vi "Multiple Chassis Synchronization - Scopes Synchronized with TCLK.vi"() -> ()   [LabVIEW 2026]
uses:
  SubVIs/NI SYNC Abstraction/Lib/Trigger Routing.ctl
  SubVIs/NI SYNC Abstraction/Lib/Clock Routing.ctl
  <instrlib>/niScope/Controls/niScope export destinations.ctl
  Types/MyState.ctl
  <instrlib>/niScope/Controls/niScope input clock source.ctl
  Types/MyVariables.ctl
  <instrlib>/niScope/Controls/niScope exportable signals.ctl
  <instrlib>/niFgen/niFgen.llb/niFgen Output Mode.ctl
  <instrlib>/niScope/Configure/Trigger/niScope Configure Trigger Edge.vi
  <instrlib>/niScope/Configure/Trigger/niScope Configure Trigger Digital.vi
  <instrlib>/niSync/niSync.llb/niSync Initialize (IVI).vi
  SubVIs/NI SYNC Abstraction/Lib/Connect Clock Terminals-Array.vi
  SubVIs/NI SYNC Abstraction/Lib/Connect Clock Terminals.vi
  SubVIs/NI SYNC Abstraction/Lib/Connect Trigger Terminals-Array.vi
  SubVIs/NI SYNC Abstraction/Lib/Connect Trigger Terminals.vi
  SubVIs/NI SYNC Abstraction/Lib/Disonnect Trigger Terminals-Array.vi
  SubVIs/NI SYNC Abstraction/Lib/Disonnect Trigger Terminals.vi
  <instrlib>/niScope/Acquire/Fetch/niScope Fetch Cluster.vi
  SubVIs/NI SYNC Abstraction/Lib/Disconnect Clock Terminals-Array.vi
  SubVIs/NI SYNC Abstraction/Lib/Disconnect Clock Terminals.vi
  <resource>/objmgr/sessionReference.rc
  <vilib>/ptbypt/NI_PtbyPt.lvlib
panel:
  in  "Tab Control":T1(tab)
  in  "Master.Scope":refnum<k15>="PXI1_SCOPE1"
  in  "Rest.Scopes":refnum<k15>[](array[refnum])=["PXI2_SCOPE2"]
  in  "Master.6674T_1":refnum<k15>="PXI1_MasterSync"
  in  "Rest.6674T_1":refnum<k15>="PXI2_SlaveSync"
  in  "FGEN.Ref":refnum<k15>="PXI1_FGEN1"
  in  "Routing":T2(tab)
  in  "Rest.In --> Clk10":T3={"Source Terminal"="ClkIn", "Destination Terminal"="PXI_Clk10_In"}
  in  "Master.In --> Clk10":T3={"Source Terminal"="ClkIn", "Destination Terminal"="PXI_Clk10_In"}
  in  "Master.Clock --> Out":T3={"Source Terminal"="Oscillator", "Destination Terminal"="ClkOut"}
  in  "Rest.PFI --> Ref Trigger":T4={"Source"="PFI0", "Destination"="PXI_Trig0", "Synchronization Clock"="SyncClkAsync"}
  in  "Master.Ref Trigger --> PFI":T4={"Source"="PXI_Trig0", "Destination"="PFI0", "Synchronization Clock"="SyncClkAsync"}
  in  "Master.Ref Trigger Export":T5="VAL_RTSI_0"
  in  "Rest.Ref Trigger Source":T5="VAL_RTSI_0"
  in  "Rest.Start Trigger Source":T5="VAL_RTSI_1"
  in  "Rest.PFI --> Start Trigger":T4={"Source"="PFI1", "Destination"="PXI_Trig1", "Synchronization Clock"="SyncClkAsync"}
  in  "Master.Start Trigger --> PFI":T4={"Source"="PXI_Trig1", "Destination"="PFI2", "Synchronization Clock"="SyncClkAsync"}
  in  "Master.Start Trigger Export":T5="VAL_RTSI_1"
  in  "Rest.Sync Pulse Source":string(combo)="PXI_Trig2"
  in  "Rest.PFI --> Sync Pulse Source":T4={"Source"="PFI1", "Destination"="PXI_Trig2", "Synchronization Clock"="SyncClkAsync"}
  in  "Master.PFI --> Sync Pulse Source":T4={"Source"="PFI1", "Destination"="PXI_Trig2", "Synchronization Clock"="SyncClkAsync"}
  in  "Master.Sync Pulse Export --> PFI":T4={"Source"="PXI_Trig3", "Destination"="PFI2", "Synchronization Clock"="SyncClkFullSpeed"}
  in  "Master.Sync Pulse Export":string(combo)="PXI_Trig3"
  in  "Master.Sync Pulse Source":string(combo)="PXI_Trig2"
  in  "Enable Cal?":bool
  in  "Calibration Iterations":i32=10
  in  "Scope 2 tCLK Delay":dbl format="%#_13p"
  in  "Scope 1 tCLK Delay":dbl format="%#_13p"
  out "Cal Iteration Delays":dbl[](array[numeric]) format="%#_p"
  out "Average Delay":dbl format="%.5p"
  out "Standard Deviation":dbl format="%0.2p"
  out "Waveform Graph":T6(graph)
  out "Sample Offset":dbl
  out "error out":errorcluster
  out "Offset Time (s)":dbl format="%#_p"
  # "Scope"
  # "Sync"
  # "Master"
  # "Ref Trigger Export"
  # "Start Trigger Export"
  # "Sync Pulse Source"
  # "Sync Pulse Export"
  # "Sync"
  # "Scope"
  # "Rest"
  # "Ref Trigger Source"
  # "Start Trigger Source"
  # "Sync Pulse Source"
  # "None"
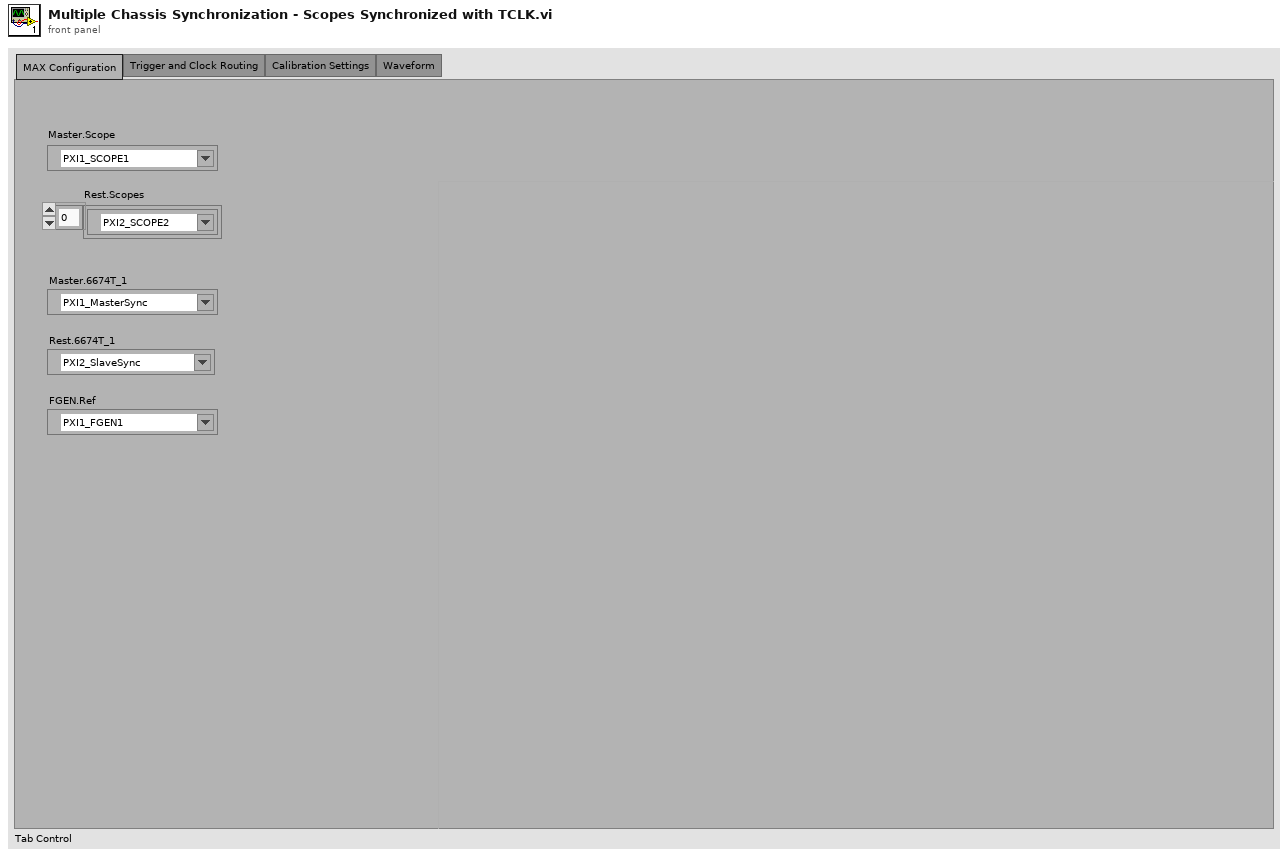
[diagram p1: front panel]
types:
  T1 = enum32{"MAX Configuration", "Trigger and Clock Routing", "Calibration Settings", "Waveform"}
  T2 = enum32{"Clock Routing", "Reference Trigger", "Start Trigger", "Sync Pulse"}
  T3 = typedef "Clock Routing.ctl" = cluster{"Source Terminal":string, "Destination Terminal":string}
  T4 = typedef "Trigger Routing.ctl" = cluster{"Source":string, "Destination":string, "Synchronization Clock":string}
  T5 = typedef "niScope export destinations.ctl" = string
  T6 = cluster{"relativeInitialX":dbl, "xIncrement":dbl, "wfm":dbl[]}[]
  T7 = typedef "MyState.ctl" = enum16{"Initialize", "SCOPE: Config.Master", "SCOPE: Config.Rest", "SYNC: Device.Init", "SYNC: ConnectClock.Master", "SYNC: ConnectClock.Rest", "SYNC: ConnectSyncPulse.Master", "SYNC: ConnectSyncPulse.Rest", "SYNC: ConnectRefTrigger.Master", "SYNC: ConnectRefTrigger.Rest", "TCLK: Config.Master", "TCLK: Config.Rest", "TCLK: ApplyManualCalibration", "TCLK: SendSyncPulse", "SYNC: DisconnectSyncPulse.Master", "SYNC: DisconnectSyncPulse.Rest", "SYNC: ConnectStartTrigger.Master", "SYNC: ConnectStartTrigger.Rest", "TCLK: Commit", "FGEN: StartSquareWave", "SCOPE: Acquire", "FGEN: StopSquareWave", "SYNC: DisconnectStartTrigger.Master", "SYNC: DisconnectStartTrigger.Rest", "SYNC: DisconnectRefTrigger.Master", "SYNC: DisconnectRefTrigger.Rest", "SYNC: DisconnectClock.Master", "SYNC: DisconnectClock.Rest", "Shutdown"}
  T8 = typedef "MyVariables.ctl" = cluster{"Master":cluster{"TimeSync.Ref":refnum<k15>, "TCLK.Ref":refnum<k20>, "Clock":cluster{"Clock --> Out":T3, "In --> Clk10":T3}, "Sync Pulse":cluster{"Sync Pulse Export":string, "Sync Pulse Export --> PFI":T4, "PFI --> Sync Pulse Source":T4, "Sync Pulse Source":string}, "Start Trigger":cluster{"Start Trigger Export":T5, "Start Trigger --> PFI":T4}, "Scope.Ref":refnum<k15>, "Ref Trigger":cluster{"Ref Trigger Export":T5, "Ref Trigger --> PFI":T4}}, "Rest":cluster{"TimeSync.Ref":refnum<k15>, "TCLK.Refs":refnum<k20>[], "Clock":cluster{"In --> Clk10":T3}, "Sync Pulse":cluster{"PFI --> Sync Pulse Source":T4, "Sync Pulse Source":string}, "Start Trigger":cluster{"PFI --> Start Trigger":T4, "Start Trigger Source":T5}, "Scope.Refs":refnum<k15>[], "Ref Trigger":cluster{"PFI --> Ref Trigger":T4, "Ref Trigger Source":T5}}, "FGEN.Ref":refnum<k15>}
  T9 = typedef "niScope input clock source.ctl" = u16
  T10 = typedef "niScope exportable signals.ctl" = u16
  T11 = typedef "niFgen Output Mode.ctl" = u32
  T12 = cluster{"relativeInitialX":dbl, "xIncrement":dbl, "wfm":dbl[]}
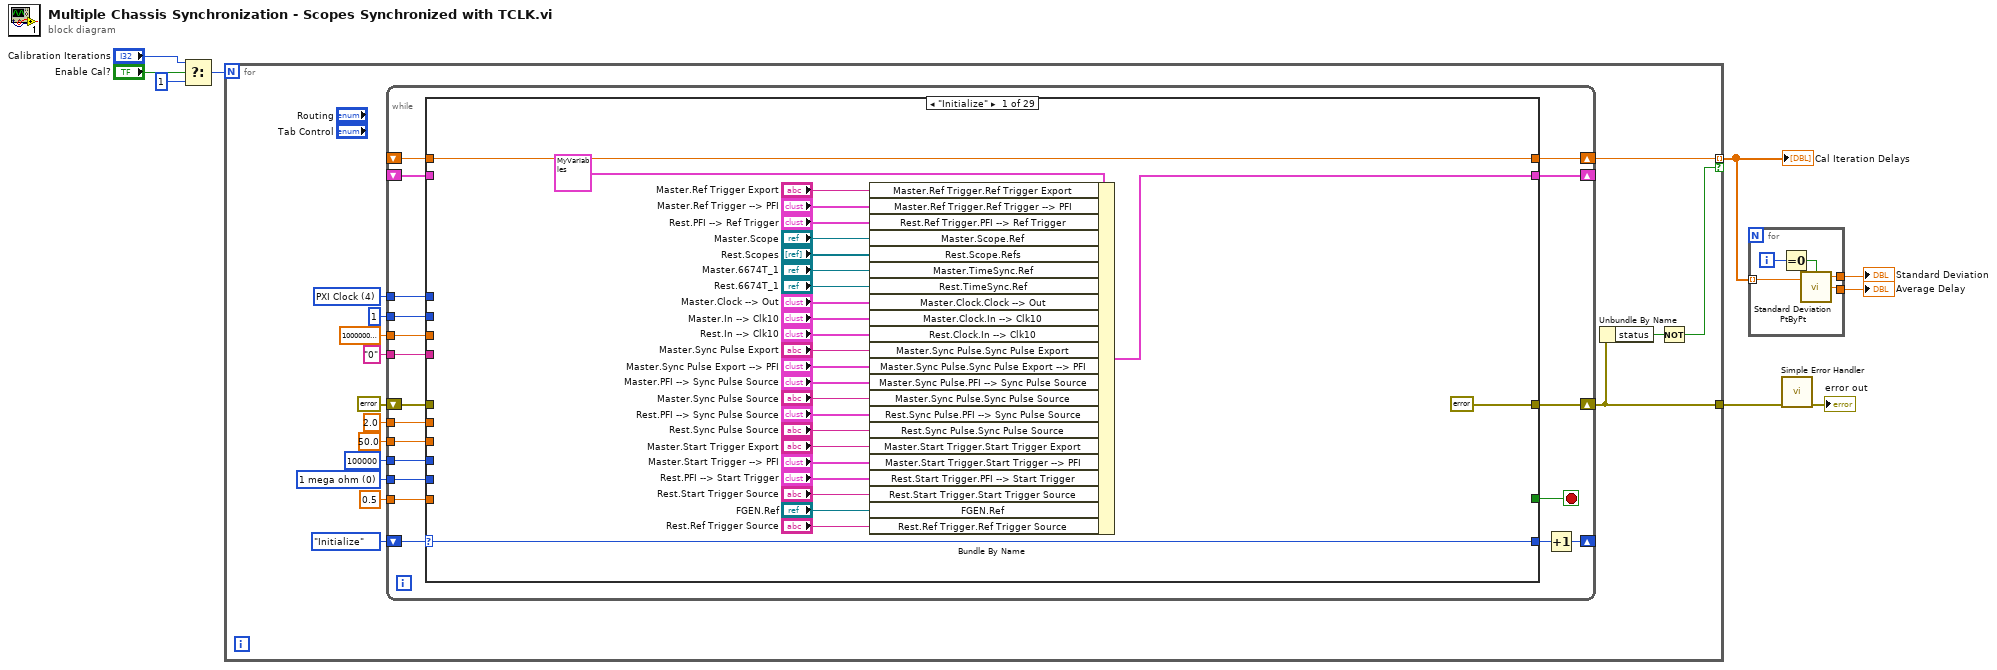
[diagram p0: block diagram]
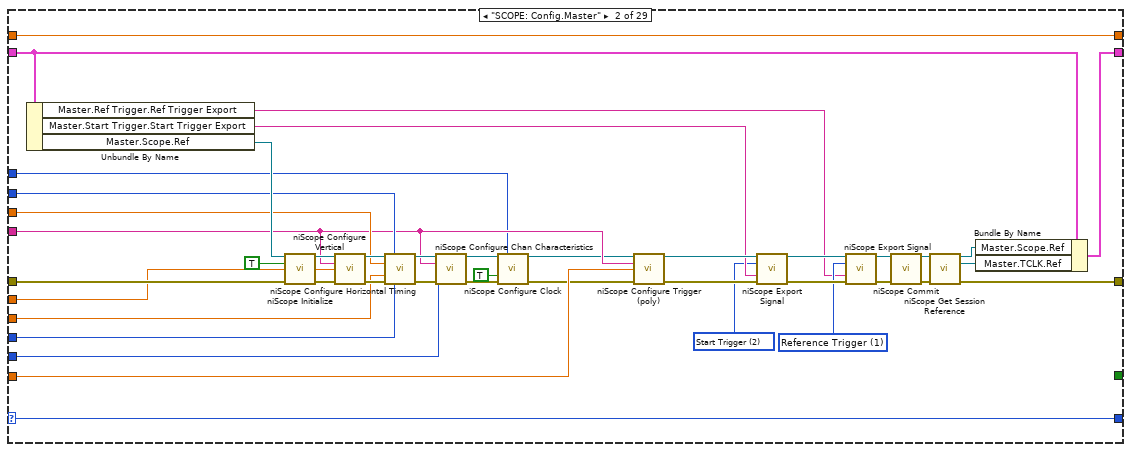
[diagram p2: hidden frame]
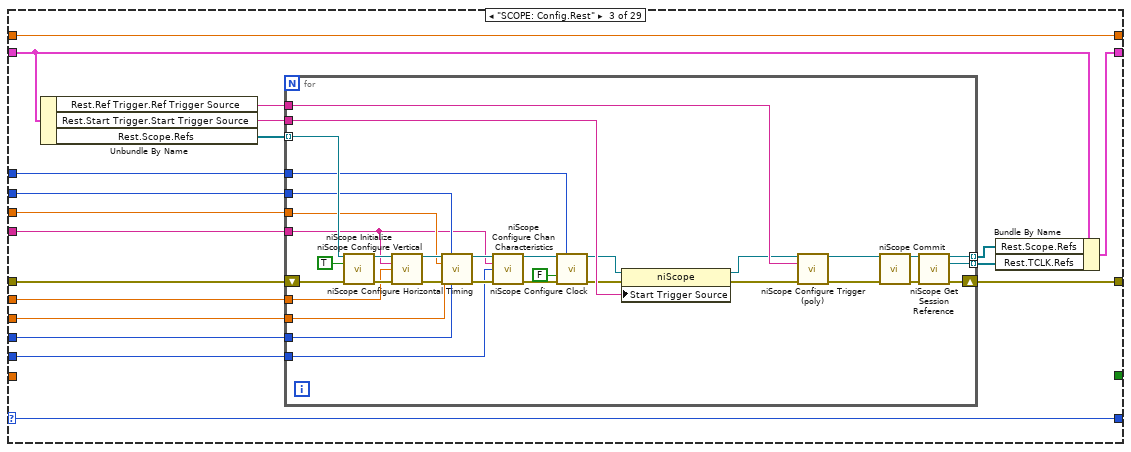
[diagram p3: hidden frame]
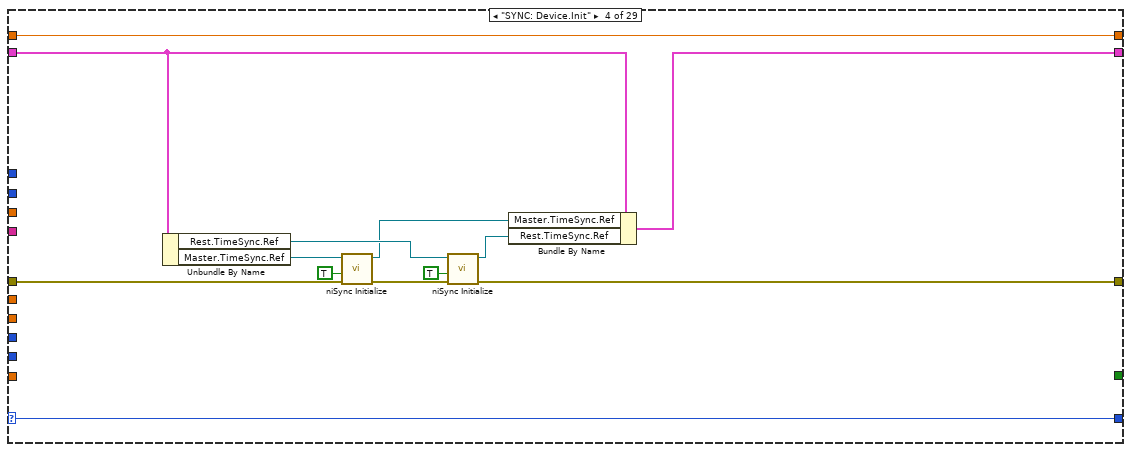
[diagram p4: hidden frame]
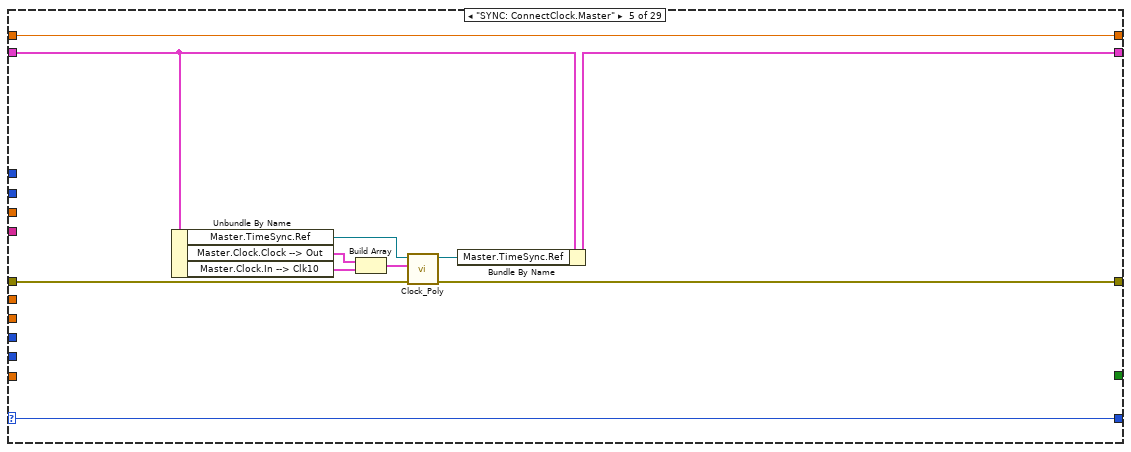
[diagram p5: hidden frame]
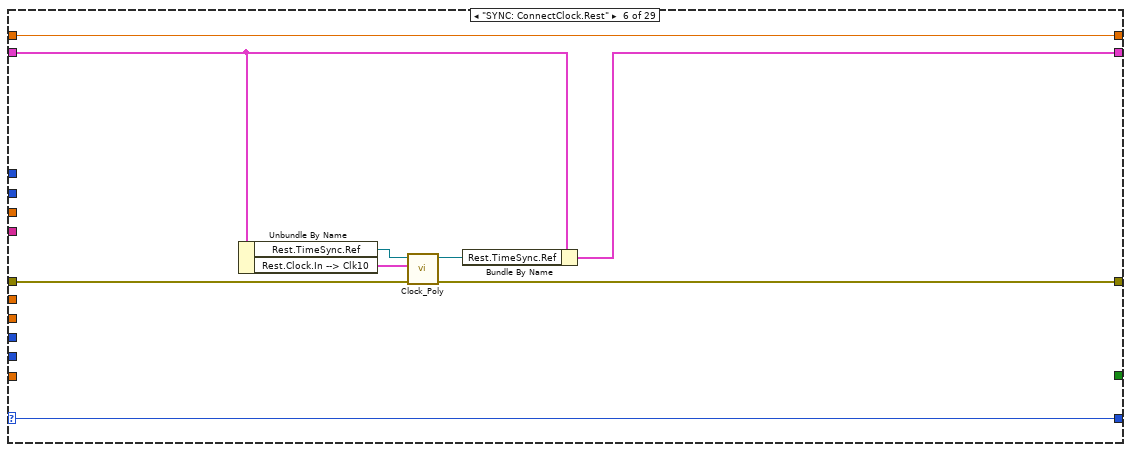
[diagram p6: hidden frame]
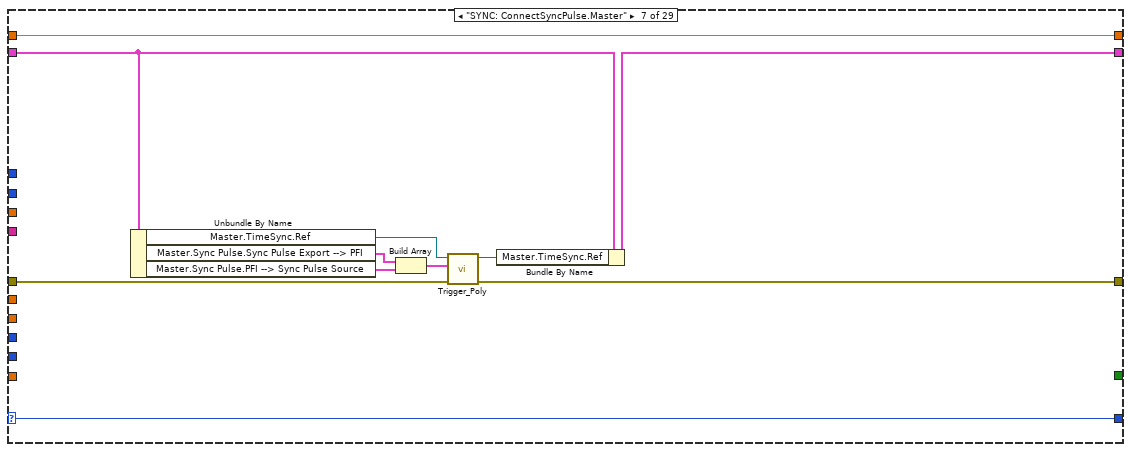
[diagram p7: hidden frame]
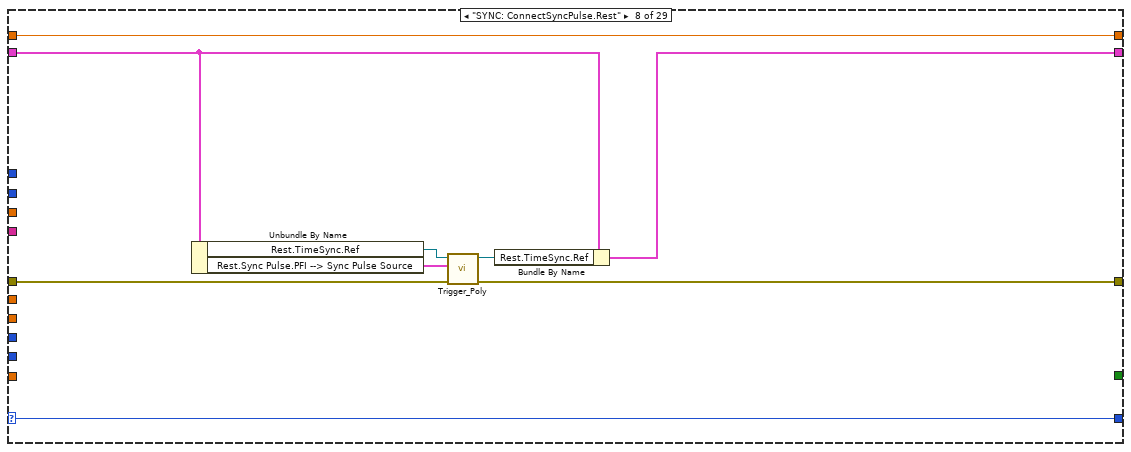
[diagram p8: hidden frame]
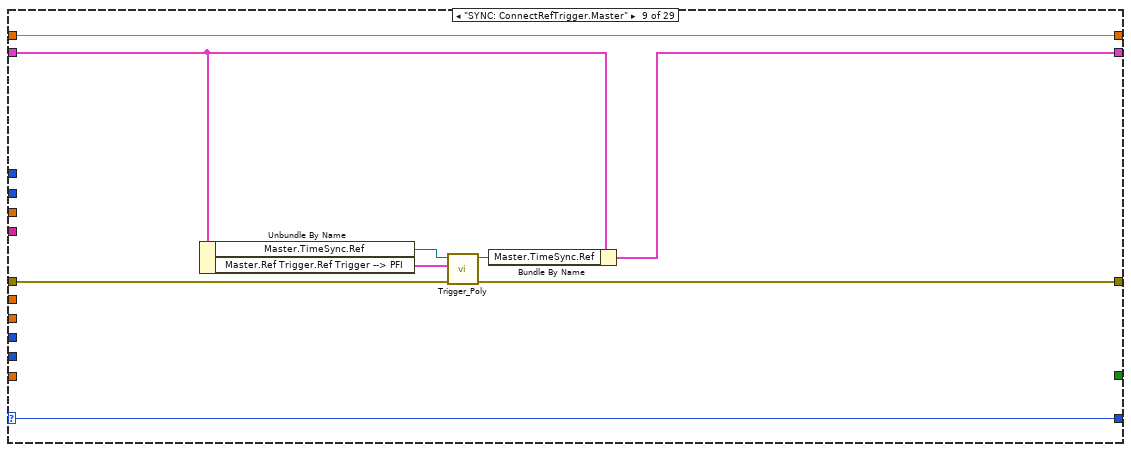
[diagram p9: hidden frame]
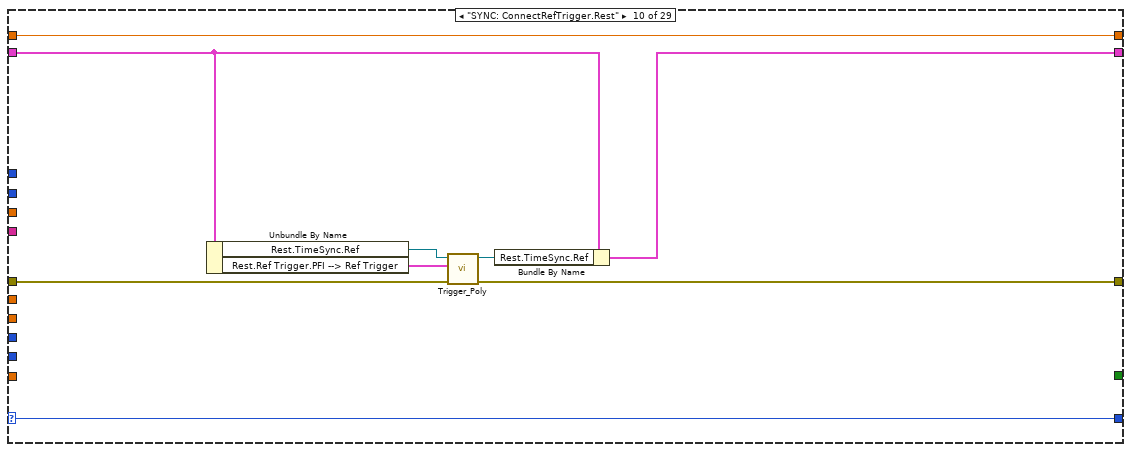
[diagram p10: hidden frame]
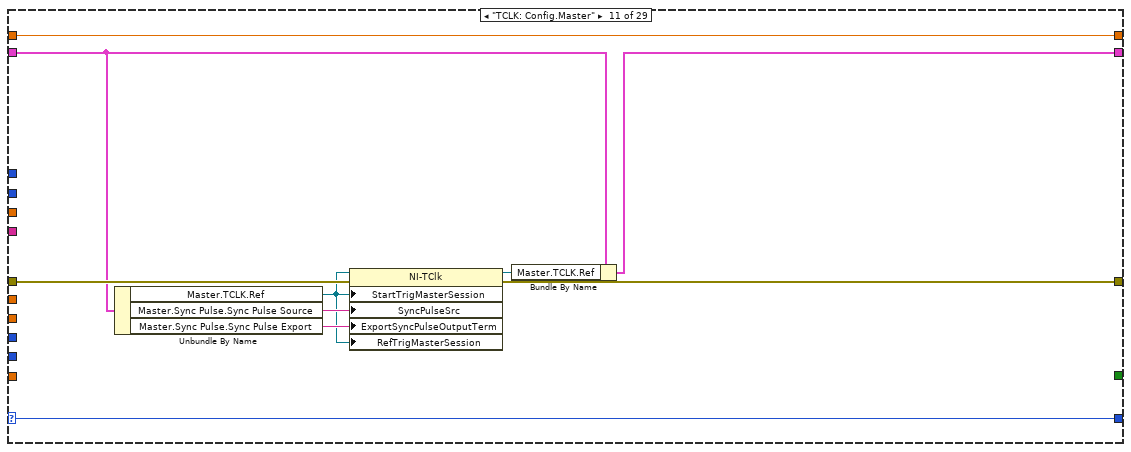
[diagram p11: hidden frame]
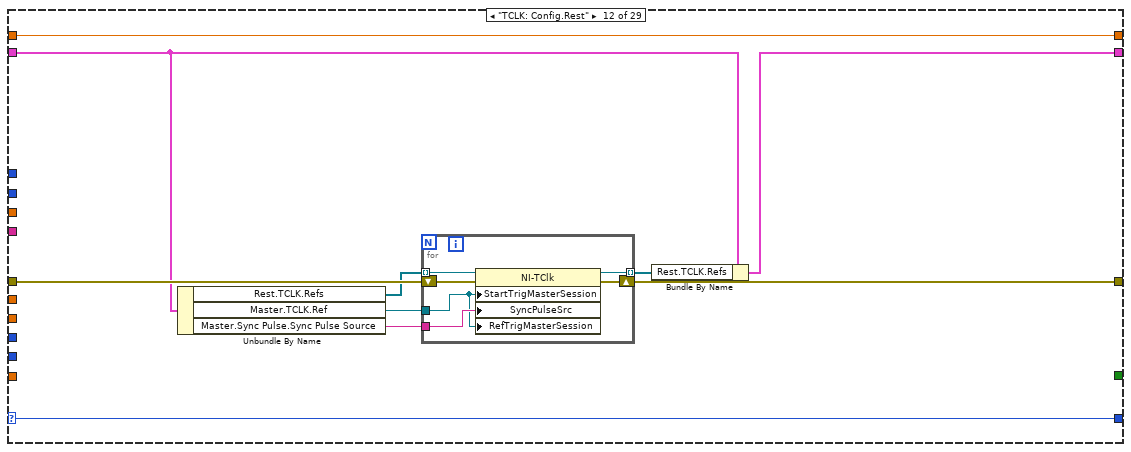
[diagram p12: hidden frame]
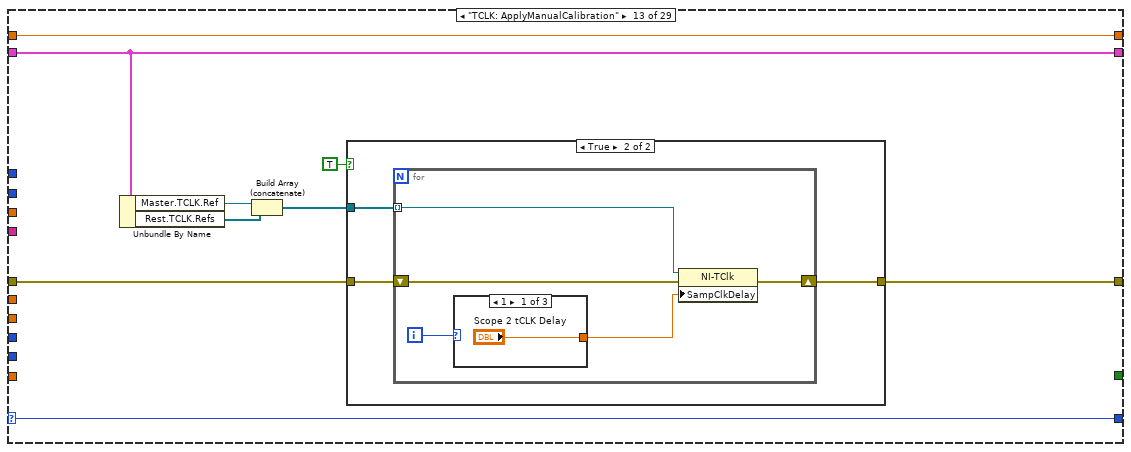
[diagram p13: hidden frame]
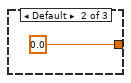
[diagram p15: hidden frame]
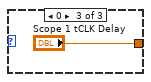
[diagram p16: hidden frame]
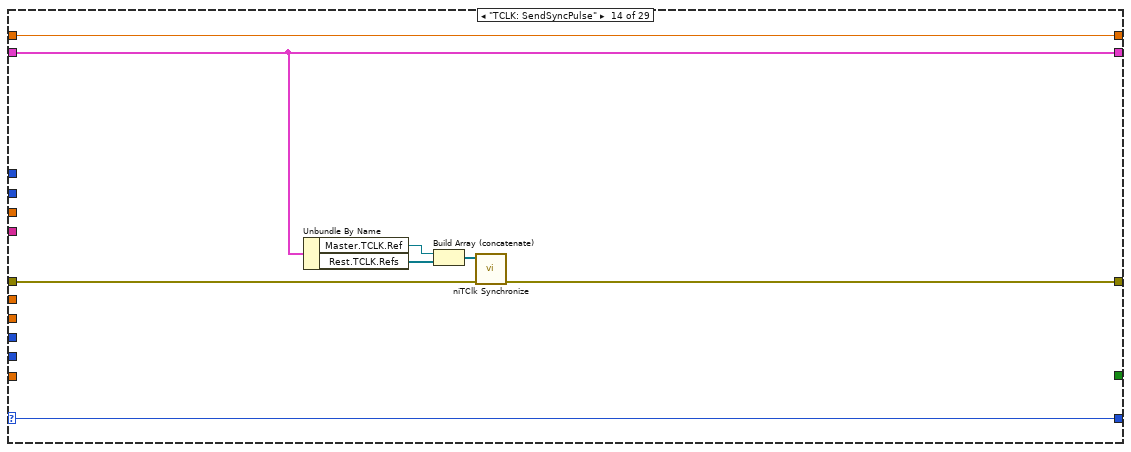
[diagram p17: hidden frame]
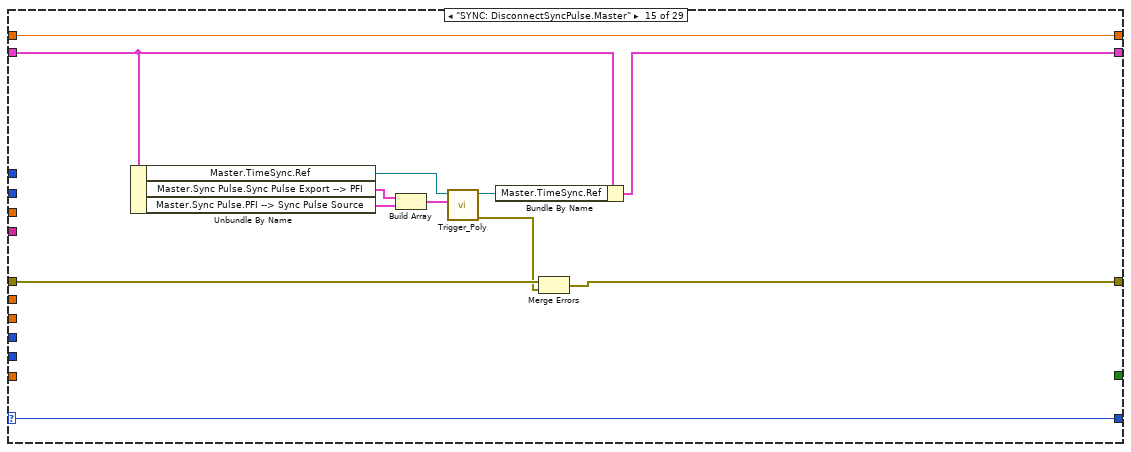
[diagram p18: hidden frame]
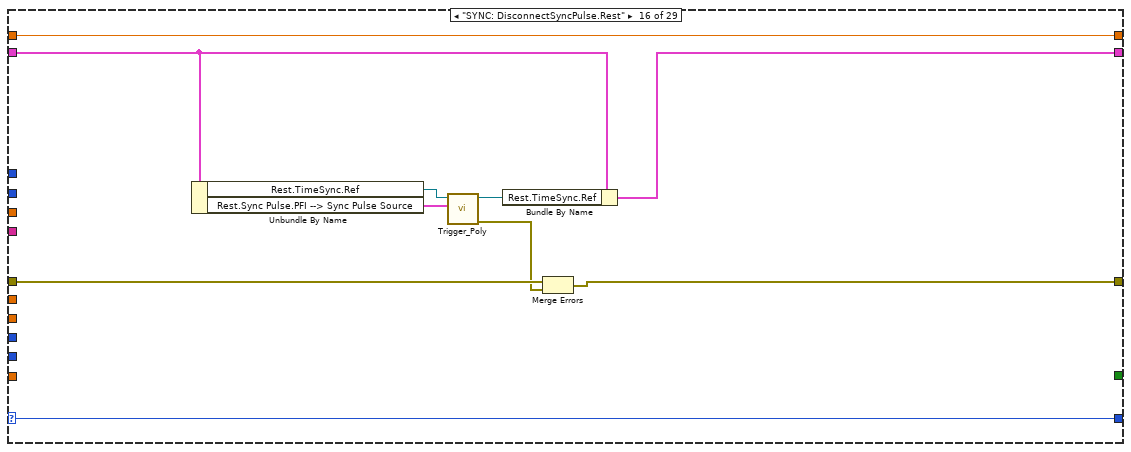
[diagram p19: hidden frame]
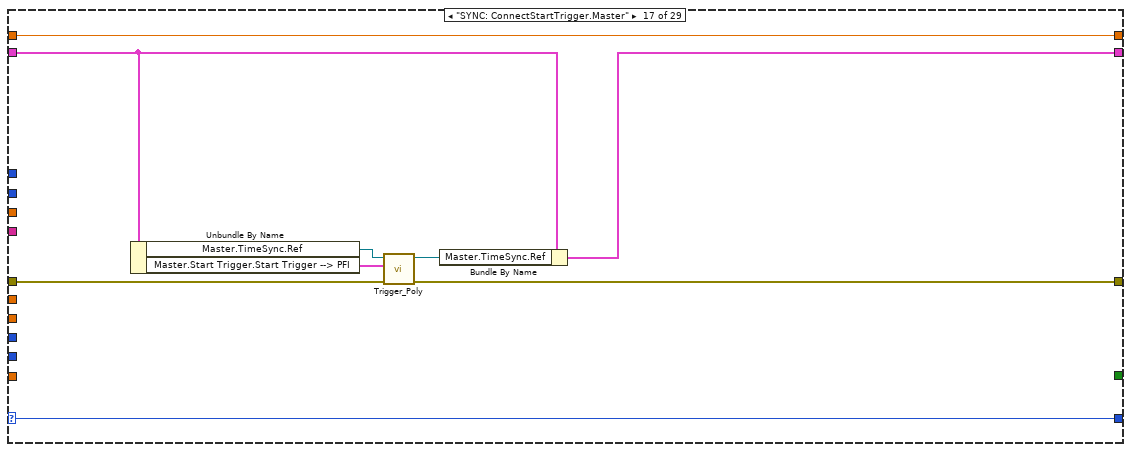
[diagram p20: hidden frame]
diagram:
  n1 = Select(t="Calibration Iterations", s="Enable Cal?", f=1) -> (s? t:f=w4:i32)
  n2 = for {
    N: w4 -> [_]
    tunnel: [w13] -> w9
    tunnel: [w14] -> w3 mode=indexing if=w11
    w10 = T9 4 items=["None"=0, "RTSI Clock"=1, "PFI 0"=6, "PFI 1"=2, "PFI 2"=3, "PXI Clock"=4, "External"=5, "Clock In"=7] ("input clock source")
    w18 = u32 0 items=["1 mega ohm"=0, "50 ohms"=2] ("input impedance")
    n3 = while {
      shift-right: [w36] -> _
      shift-left: MyState."Initialize" -> [w43]
      shift-right: [w42] -> _
      shift-left: _ -> [w41]
      shift-right: [w39] -> w13
      shift-left: errorcluster {"status"=FALSE, "code"=0, "source"=""} ("error out") -> [w40]
      tunnel: 100000000.0 ("min sample rate") -> [w35]
      tunnel: 100000 ("min record length") -> [w34]
      tunnel: 2.0 ("vertical offset") -> [w33]
      tunnel: 50.0 ("reference position") -> [w32]
      tunnel: w18 -> [w31]
      tunnel: 1 ("number of records") -> [w30]
      tunnel: "0" ("channels") -> [w29]
      tunnel: 0.5 ("trigger level") -> [w28]
      shift-right: [w27] -> w14
      shift-left: _ -> [w26]
      tunnel: w10 -> [w25]
      stop <- w37 stop-if-true
      n4 = case shown="\"Initialize\"" w43 {
        selector: w43 -> [w53 w112 w131 w167 w179 w191 w199 w211 w220 w229 w245 w255 w270 w290 w295 w308 w315 w324 w338 w347 w380 w392 w404 w415 w425 w435 w444 w457 w464]
        tunnel: [w54 w110 w130 w171 w187 w196 w207 w216 w225 w234 w238 w248 w269 w287 w301 w311 w320 w329 w335 w344 w377 w397 w408 w418 w428 w438 w450 w460 w475] -> w42
        tunnel: w41 -> [_ w96 w127 w172 w188 w197 w208 w217 w226 w235 w240 w250 w269 w287 w302 w312 w321 w330 w335 w346 w377 w397 w409 w419 w429 w439 w451 w461 w475]
        tunnel: [w53 w112 w131 w167 w179 w191 w199 w211 w220 w229 w245 w255 w270 w290 w295 w308 w315 w324 w338 w347 w380 w392 w404 w415 w425 w435 w444 w457 w464] -> w38
        tunnel: [errorcluster {"status"=FALSE, "code"=0, "source"=""} ("error out") w109 w129 w168 w184 w193 w204 w213 w222 w231 w243 w253 w266 w288 w292 w304 w317 w326 w332 w348 w374 w393 w402 w413 w421 w432 w442 w454 w465] -> w39
        tunnel: w40 -> [_ w98 w128 w166 w180 w192 w200 w212 w221 w230 w244 w254 w267 w289 w294 w306 w316 w325 w333 w349 w379 w394 w401 w411 w423 w431 w443 w455 w468]
        tunnel: [_ _ _ _ _ _ _ _ _ _ _ _ _ _ _ _ _ _ _ _ _ _ _ _ _ _ _ _ TRUE] -> w37
        tunnel: w35 -> [_ w84 w120 _ _ _ _ _ _ _ _ _ _ _ _ _ _ _ _ _ w365 _ _ _ _ _ _ _ _]
        tunnel: w34 -> [_ w83 w116 _ _ _ _ _ _ _ _ _ _ _ _ _ _ _ _ _ w366 _ _ _ _ _ _ _ _]
        tunnel: w33 -> [_ w82 w118 _ _ _ _ _ _ _ _ _ _ _ _ _ _ _ _ _ _ _ _ _ _ _ _ _ _]
        tunnel: w32 -> [_ w81 w117 _ _ _ _ _ _ _ _ _ _ _ _ _ _ _ _ _ _ _ _ _ _ _ _ _ _]
        tunnel: w31 -> [_ w80 w115 _ _ _ _ _ _ _ _ _ _ _ _ _ _ _ _ _ _ _ _ _ _ _ _ _ _]
        tunnel: w30 -> [_ w79 w121 _ _ _ _ _ _ _ _ _ _ _ _ _ _ _ _ _ _ _ _ _ _ _ _ _ _]
        tunnel: w29 -> [_ w78 w119 _ _ _ _ _ _ _ _ _ _ _ _ _ _ _ _ _ _ _ _ _ _ _ _ _ _]
        tunnel: w28 -> [_ w77 _ _ _ _ _ _ _ _ _ _ _ _ _ _ _ _ _ w342 w362 _ _ _ _ _ _ _ _]
        tunnel: [w45 w76 w114 w165 w178 w189 w198 w209 w218 w227 w236 w246 w262 w283 w291 w303 w313 w322 w331 w339 w361 w391 w400 w410 w420 w430 w440 w452 w462] -> w27
        tunnel: w26 -> [w45 w76 w114 w165 w178 w189 w198 w209 w218 w227 w236 w246 w262 w283 w291 w303 w313 w322 w331 w339 _ w391 w400 w410 w420 w430 w440 w452 w462]
        tunnel: w25 -> [_ w72 w113 _ _ _ _ _ _ _ _ _ _ _ _ _ _ _ _ _ _ _ _ _ _ _ _ _ _]
        frame "Initialize" {
          n5 = Bundle By Name(cluster=T8 {"Master"={"TimeSync.Ref"="PXI_Trig0", "TCLK.Ref"=refnum, "Clock"={"Clock --> Out"={"Source Terminal"="Oscillator", "Destination Terminal"="ClkOut"}, "In --> Clk10"={"Source Terminal"="ClkIn", "Destination Terminal"="PXI_Clk10_In"}}, "Sync Pulse"={"Sync Pulse Export"="SyncClkFullSpeed", "Sync Pulse Export --> PFI"={"Source"="ClkIn", "Destination"="PXI_Clk10_In", "Synchronization Clock"="SyncClkAsync"}, "PFI --> Sync Pulse Source"={"Source"="PXI_Trig2", "Destination"="PFI2", "Synchronization Clock"="SyncClkAsync"}, "Sync Pulse Source"="PFI1"}, "Start Trigger"={"Start Trigger Export"="PXI_Trig2", "Start Trigger --> PFI"={"Source"="SyncClkAsync", "Destination"="VAL_RTSI_2", "Synchronization Clock"=""}}, "Scope.Ref"="", "Ref Trigger"={"Ref Trigger Export"="VAL_RTSI_2", "Ref Trigger --> PFI"={"Source"="PXI_Trig3", "Destination"="PFI0", "Synchronization Clock"="SyncClkAsync"}}}, "Rest"={"TimeSync.Ref"="", "TCLK.Refs"=[], "Clock"={"In --> Clk10"={"Source Terminal"="PXI_Trig0", "Destination Terminal"="PFI2"}}, "Sync Pulse"={"PFI --> Sync Pulse Source"={"Source"="PFI1", "Destination"="PXI_Trig1", "Synchronization Clock"="SyncClkAsync"}, "Sync Pulse Source"="PXI_Trig1"}, "Start Trigger"={"PFI --> Start Trigger"={"Source"="PFI1", "Destination"="PXI_Trig2", "Synchronization Clock"="SyncClkAsync"}, "Start Trigger Source"="VAL_RTSI_2"}, "Scope.Refs"=[], "Ref Trigger"={"PFI --> Ref Trigger"={"Source"="PFI0", "Destination"="PXI_Trig3", "Synchronization Clock"="SyncClkAsync"}, "Ref Trigger Source"="VAL_RTSI_3"}}, "FGEN.Ref"=""} ("Routes"), "Master.Ref Trigger.Ref Trigger Export"="Master.Ref Trigger Export", "Master.Ref Trigger.Ref Trigger --> PFI"="Master.Ref Trigger --> PFI", "Rest.Ref Trigger.PFI --> Ref Trigger"="Rest.PFI --> Ref Trigger", "Master.Scope.Ref"="Master.Scope", "Rest.Scope.Refs"="Rest.Scopes", "Master.TimeSync.Ref"="Master.6674T_1", "Rest.TimeSync.Ref"="Rest.6674T_1", "Master.Clock.Clock --> Out"="Master.Clock --> Out", "Master.Clock.In --> Clk10"="Master.In --> Clk10", "Rest.Clock.In --> Clk10"="Rest.In --> Clk10", "Master.Sync Pulse.Sync Pulse Export"="Master.Sync Pulse Export", "Master.Sync Pulse.Sync Pulse Export --> PFI"="Master.Sync Pulse Export --> PFI", "Master.Sync Pulse.PFI --> Sync Pulse Source"="Master.PFI --> Sync Pulse Source", "Master.Sync Pulse.Sync Pulse Source"="Master.Sync Pulse Source", "Rest.Sync Pulse.PFI --> Sync Pulse Source"="Rest.PFI --> Sync Pulse Source", "Rest.Sync Pulse.Sync Pulse Source"="Rest.Sync Pulse Source", "Master.Start Trigger.Start Trigger Export"="Master.Start Trigger Export", "Master.Start Trigger.Start Trigger --> PFI"="Master.Start Trigger --> PFI", "Rest.Start Trigger.PFI --> Start Trigger"="Rest.PFI --> Start Trigger", "Rest.Start Trigger.Start Trigger Source"="Rest.Start Trigger Source", "FGEN.Ref"="FGEN.Ref", "Rest.Ref Trigger.Ref Trigger Source"="Rest.Ref Trigger Source") -> (w54:T8)
        }
        frame "SCOPE: Config.Master" {
          w86 = T10 1 items=["None"=0, "Start Trigger"=2, "Advance Trigger"=5, "Reference Trigger"=1, "End of Record Event"=4, "End of Acquisition Event"=3, "Ready for Start Event"=7, "Ready for Advance Event"=6, "Ready for Reference Event"=10, "Reference Clock"=100, "Sample Clock"=101, "5 Volt Power"=13] ("signal")
          w91 = T10 2 items=["None"=0, "Start Trigger"=2, "Advance Trigger"=5, "Reference Trigger"=1, "End of Record Event"=4, "End of Acquisition Event"=3, "Ready for Start Event"=7, "Ready for Advance Event"=6, "Ready for Reference Event"=10, "Reference Clock"=100, "Sample Clock"=101, "5 Volt Power"=13] ("signal")
          n6 = Unbundle By Name(w96) -> ("Master.Ref Trigger.Ref Trigger Export"=w85:T5, "Master.Start Trigger.Start Trigger Export"=w95:T5, "Master.Scope.Ref"=w94:refnum<k15>)
          n7 = call <instrlib>:"niScope Initialize.vi"("resource name"=w94, "id query"=TRUE, "error in"=w98) -> ("instrument handle"=w107:refnum<k15>, "error out"=w104:errorcluster)  [unwired: 11 in]
          n8 = call <instrlib>:"niScope Configure Vertical.vi"("instrument handle"=w107, "channels"=w78, "vertical range"=w82, "error in"=w104) -> ("instrument handle out"=w106:refnum<k15>, "error out"=w103:errorcluster)  [unwired: 10 in]
          n9 = call <instrlib>:"niScope Configure Horizontal Timing.vi"("instrument handle"=w106, "number of records"=w79, "min sample rate"=w84, "reference position"=w81, "error in"=w103, "min record length"=w83) -> ("instrument handle out"=w105:refnum<k15>, "error out"=w102:errorcluster)  [unwired: 8 in]
          n10 = call <instrlib>:"niScope Configure Chan Characteristics.vi"("instrument handle"=w105, "channels"=w78, "input impedance"=w80, "error in"=w102) -> ("instrument handle out"=w101:refnum<k15>, "error out"=w74:errorcluster)  [unwired: 10 in]
          n11 = call <instrlib>:"niScope Configure Clock.vi"("instrument handle"=w101, "input clock source"=w72, "master enabled"=TRUE, "error in"=w74) -> ("instrument handle out"=w75:refnum<k15>, "error out"=w73:errorcluster)  [unwired: 10 in]
          n12 = call-poly <instrlib>:"niScope Configure Trigger (poly).vi"("instrument handle"=w75, "trigger source"=w78, "trigger level"=w77, "error in"=w73) -> ("instrument handle out"=w97:refnum<k15>, "error out"=w100:errorcluster)  [unwired: 10 in]
          n13 = call <instrlib>:"niScope Export Signal.vi"("instrument handle"=w97, "signal"=w91, "output terminal"=w95, "error in"=w100) -> ("instrument handle out"=w89:refnum<k15>, "error out"=w90:errorcluster)  [unwired: 10 in]
          n14 = call <instrlib>:"niScope Export Signal.vi"("instrument handle"=w89, "signal"=w86, "output terminal"=w85, "error in"=w90) -> ("instrument handle out"=w87:refnum<k15>, "error out"=w88:errorcluster)  [unwired: 10 in]
          n15 = call <instrlib>:"niScope Commit.vi"("instrument handle"=w87, "error in"=w88) -> ("instrument handle out"=w93:refnum<k15>, "error out"=w99:errorcluster)  [unwired: 12 in]
          n16 = call <instrlib>:"niScope Get Session Reference.vi"("instrument handle"=w93, "error in"=w99) -> ("instrument handle out"=w92:refnum<k15>, "session reference"=w111:refnum<k20>, "error out"=w109:errorcluster)  [unwired: 11 in]
          n17 = Bundle By Name(cluster=w96, "Master.Scope.Ref"=w92, "Master.TCLK.Ref"=w111) -> (w110:T8)
        }
        frame "SCOPE: Config.Rest" {
          n18 = Unbundle By Name(w127) -> ("Rest.Ref Trigger.Ref Trigger Source"=w122:T5, "Rest.Start Trigger.Start Trigger Source"=w126:T5, "Rest.Scope.Refs"=w123:refnum<k15>[])
          n19 = for {
            tunnel: w126 -> [w154]
            shift-right: [w164] -> w129
            shift-left: w128 -> [w155]
            tunnel: [w150] -> w125 mode=indexing
            tunnel: [w149] -> w124 mode=indexing
            tunnel: w123 -> [w148] mode=indexing
            tunnel: w122 -> [w147]
            tunnel: w121 -> [w144]
            tunnel: w120 -> [w143]
            tunnel: w119 -> [w142]
            tunnel: w118 -> [w141]
            tunnel: w117 -> [w140]
            tunnel: w116 -> [w139]
            tunnel: w115 -> [w138]
            tunnel: w113 -> [w132]
            n20 = call <instrlib>:"niScope Initialize.vi"("resource name"=w148, "id query"=TRUE, "error in"=w155) -> ("instrument handle"=w162:refnum<k15>, "error out"=w159:errorcluster)  [unwired: 11 in]
            n21 = call <instrlib>:"niScope Configure Vertical.vi"("instrument handle"=w162, "channels"=w142, "vertical range"=w141, "error in"=w159) -> ("instrument handle out"=w161:refnum<k15>, "error out"=w158:errorcluster)  [unwired: 10 in]
            n22 = call <instrlib>:"niScope Configure Horizontal Timing.vi"("instrument handle"=w161, "number of records"=w144, "min sample rate"=w143, "reference position"=w140, "error in"=w158, "min record length"=w139) -> ("instrument handle out"=w160:refnum<k15>, "error out"=w157:errorcluster)  [unwired: 8 in]
            n23 = call <instrlib>:"niScope Configure Chan Characteristics.vi"("instrument handle"=w160, "channels"=w142, "input impedance"=w138, "error in"=w157) -> ("instrument handle out"=w136:refnum<k15>, "error out"=w135:errorcluster)  [unwired: 10 in]
            n24 = call <instrlib>:"niScope Configure Clock.vi"("instrument handle"=w136, "input clock source"=w132, "master enabled"=FALSE, "error in"=w135) -> ("instrument handle out"=w133:refnum<k15>, "error out"=w134:errorcluster)  [unwired: 10 in]
            n25 = property class="niScope"(reference=w133, error in=w134, "Start Trigger Source"=w154) -> (reference out=w145:refnum<k15>, error out=w146:errorcluster)
            n26 = call-poly <instrlib>:"niScope Configure Trigger (poly).vi"("instrument handle"=w145, "trigger source"=w147, "error in"=w146) -> ("instrument handle out"=w152:refnum<k15>, "error out"=w153:errorcluster)  [unwired: 11 in]
            n27 = call <instrlib>:"niScope Commit.vi"("instrument handle"=w152, "error in"=w153) -> ("instrument handle out"=w151:refnum<k15>, "error out"=w156:errorcluster)  [unwired: 12 in]
            n28 = call <instrlib>:"niScope Get Session Reference.vi"("instrument handle"=w151, "error in"=w156) -> ("instrument handle out"=w149:refnum<k15>, "session reference"=w150:refnum<k20>, "error out"=w164:errorcluster)  [unwired: 11 in]
          }
          n29 = Bundle By Name(cluster=w127, "Rest.Scope.Refs"=w124, "Rest.TCLK.Refs"=w125) -> (w130:T8)
        }
        frame "SYNC: Device.Init" {
          n30 = Unbundle By Name(w172) -> ("Rest.TimeSync.Ref"=w176:refnum<k15>, "Master.TimeSync.Ref"=w177:refnum<k15>)
          n31 = call-poly <instrlib>:"niSync Initialize.vi"("error in (no error)"=w166, "reset device (F)"=TRUE, "resource name"=w177) -> ("error out"=w175:errorcluster, "instrument handle out"=w170:refnum<k15>)  [unwired: 7 in]
          n32 = call-poly <instrlib>:"niSync Initialize.vi"("error in (no error)"=w175, "reset device (F)"=TRUE, "resource name"=w176) -> ("error out"=w168:errorcluster, "instrument handle out"=w169:refnum<k15>)  [unwired: 7 in]
          n33 = Bundle By Name(cluster=w172, "Master.TimeSync.Ref"=w170, "Rest.TimeSync.Ref"=w169) -> (w171:T8)
        }
        frame "SYNC: ConnectClock.Master" {
          n34 = Unbundle By Name(w188) -> ("Master.TimeSync.Ref"=w186:refnum<k15>, "Master.Clock.Clock --> Out"=w183:T3, "Master.Clock.In --> Clk10"=w182:T3)
          n35 = Build Array(w183, w182) -> (w181:T3[])
          n36 = call-poly "Clock_Poly.vi"("error in (no error)"=w180, "Clock Routing"=w181, "instrument handle"=w186) -> ("error out"=w184:errorcluster, "instrument handle out"=w185:refnum<k15>)  [unwired: 7 in]
          n37 = Bundle By Name(cluster=w188, "Master.TimeSync.Ref"=w185) -> (w187:T8)
        }
        frame "SYNC: ConnectClock.Rest" {
          n38 = Unbundle By Name(w197) -> ("Rest.TimeSync.Ref"=w195:refnum<k15>, "Rest.Clock.In --> Clk10"=w190:T3)
          n39 = call-poly "Clock_Poly.vi"("error in (no error)"=w192, "Clock Routing"=w190, "instrument handle"=w195) -> ("error out"=w193:errorcluster, "instrument handle out"=w194:refnum<k15>)  [unwired: 7 in]
          n40 = Bundle By Name(cluster=w197, "Rest.TimeSync.Ref"=w194) -> (w196:T8)
        }
        frame "SYNC: ConnectSyncPulse.Master" {
          n41 = Unbundle By Name(w208) -> ("Master.TimeSync.Ref"=w206:refnum<k15>, "Master.Sync Pulse.Sync Pulse Export --> PFI"=w203:T4, "Master.Sync Pulse.PFI --> Sync Pulse Source"=w202:T4)
          n42 = Build Array(w203, w202) -> (w201:T4[])
          n43 = call-poly "Trigger_Poly.vi"("error in (no error)"=w200, "Routing Information"=w201, "instrument handle"=w206) -> ("error out"=w204:errorcluster, "instrument handle out"=w205:refnum<k15>)  [unwired: 7 in]
          n44 = Bundle By Name(cluster=w208, "Master.TimeSync.Ref"=w205) -> (w207:T8)
        }
        frame "SYNC: ConnectSyncPulse.Rest" {
          n45 = Unbundle By Name(w217) -> ("Rest.TimeSync.Ref"=w215:refnum<k15>, "Rest.Sync Pulse.PFI --> Sync Pulse Source"=w210:T4)
          n46 = call-poly "Trigger_Poly.vi"("error in (no error)"=w212, "Routing Information"=w210, "instrument handle"=w215) -> ("error out"=w213:errorcluster, "instrument handle out"=w214:refnum<k15>)  [unwired: 7 in]
          n47 = Bundle By Name(cluster=w217, "Rest.TimeSync.Ref"=w214) -> (w216:T8)
        }
        frame "SYNC: ConnectRefTrigger.Master" {
          n48 = Unbundle By Name(w226) -> ("Master.TimeSync.Ref"=w224:refnum<k15>, "Master.Ref Trigger.Ref Trigger --> PFI"=w219:T4)
          n49 = call-poly "Trigger_Poly.vi"("error in (no error)"=w221, "Routing Information"=w219, "instrument handle"=w224) -> ("error out"=w222:errorcluster, "instrument handle out"=w223:refnum<k15>)  [unwired: 7 in]
          n50 = Bundle By Name(cluster=w226, "Master.TimeSync.Ref"=w223) -> (w225:T8)
        }
        frame "SYNC: ConnectRefTrigger.Rest" {
          n51 = Unbundle By Name(w235) -> ("Rest.TimeSync.Ref"=w233:refnum<k15>, "Rest.Ref Trigger.PFI --> Ref Trigger"=w228:T4)
          n52 = call-poly "Trigger_Poly.vi"("error in (no error)"=w230, "Routing Information"=w228, "instrument handle"=w233) -> ("error out"=w231:errorcluster, "instrument handle out"=w232:refnum<k15>)  [unwired: 7 in]
          n53 = Bundle By Name(cluster=w235, "Rest.TimeSync.Ref"=w232) -> (w234:T8)
        }
        frame "TCLK: Config.Master" {
          n54 = Unbundle By Name(w240) -> ("Master.TCLK.Ref"=w237:refnum<k20>, "Master.Sync Pulse.Sync Pulse Source"=w242:string, "Master.Sync Pulse.Sync Pulse Export"=w241:string)
          n55 = property class="NI-TClk"(reference=w237, error in=w244, "StartTrigMasterSession"=w237, "SyncPulseSrc"=w242, "ExportSyncPulseOutputTerm"=w241, "RefTrigMasterSession"=w237) -> (reference out=w239:refnum<k20>, error out=w243:errorcluster)
          n56 = Bundle By Name(cluster=w240, "Master.TCLK.Ref"=w239) -> (w238:T8)
        }
        frame "TCLK: Config.Rest" {
          n57 = Unbundle By Name(w250) -> ("Rest.TCLK.Refs"=w252:refnum<k20>[], "Master.TCLK.Ref"=w247:refnum<k20>, "Master.Sync Pulse.Sync Pulse Source"=w251:string)
          n58 = for {
            tunnel: w252 -> [w259] mode=indexing
            tunnel: w251 -> [w258]
            tunnel: [w257] -> w249 mode=indexing
            tunnel: w247 -> [w256]
            shift-right: [w260] -> w253
            shift-left: w254 -> [w261]
            n59 = property class="NI-TClk"(reference=w259, error in=w261, "StartTrigMasterSession"=w256, "SyncPulseSrc"=w258, "RefTrigMasterSession"=w256) -> (reference out=w257:refnum<k20>, error out=w260:errorcluster)
          }
          n60 = Bundle By Name(cluster=w250, "Rest.TCLK.Refs"=w249) -> (w248:T8)
        }
        frame "TCLK: ApplyManualCalibration" {
          n61 = Unbundle By Name(w269) -> ("Master.TCLK.Ref"=w265:refnum<k20>, "Rest.TCLK.Refs"=w264:refnum<k20>[])
          n62 = Build Array (concatenate)(w265, w264) -> (w263:refnum<k20>[])
          n63 = case shown="True" TRUE {
            tunnel: w267 -> [w271 w274]
            tunnel: [w271 w273] -> w266
            tunnel: w263 -> [_ w272]
            frame False {
            }
            frame True {
              n64 = for {
                shift-right: [w277] -> w273
                shift-left: w274 -> [w278]
                tunnel: w272 -> [w275] mode=indexing
                i -> [w279]
                n65 = case shown="1" w279 {
                  tunnel: ["Scope 2 tCLK Delay" 0.0 ("delay") "Scope 1 tCLK Delay"] -> w276
                  frame 1 {
                  }
                  frame Default {
                  }
                  frame 0 {
                  }
                }
                n66 = property class="NI-TClk"(reference=w275, error in=w278, "SampClkDelay"=w276) -> (error out=w277:errorcluster)  [unwired: 1 out]
              }
            }
          }
        }
        frame "TCLK: SendSyncPulse" {
          n67 = Unbundle By Name(w287) -> ("Master.TCLK.Ref"=w286:refnum<k20>, "Rest.TCLK.Refs"=w285:refnum<k20>[])
          n68 = Build Array (concatenate)(w286, w285) -> (w284:refnum<k20>[])
          n69 = call <instrlib>:"niTClk Synchronize.vi"("error in (no error)"=w289, "sessions"=w284) -> ("error out"=w288:errorcluster)  [unwired: 8 in, 1 out]
        }
        frame "SYNC: DisconnectSyncPulse.Master" {
          n70 = Unbundle By Name(w302) -> ("Master.TimeSync.Ref"=w300:refnum<k15>, "Master.Sync Pulse.Sync Pulse Export --> PFI"=w298:T4, "Master.Sync Pulse.PFI --> Sync Pulse Source"=w297:T4)
          n71 = Build Array(w298, w297) -> (w296:T4[])
          n72 = call-poly "Trigger_Poly.vi"("Routing Information"=w296, "instrument handle"=w300) -> ("error out"=w293:errorcluster, "instrument handle out"=w299:refnum<k15>)  [unwired: 8 in]
          n73 = Bundle By Name(cluster=w302, "Master.TimeSync.Ref"=w299) -> (w301:T8)
          n74 = Merge Errors(w294, w293) -> (w292:errorcluster)
        }
        frame "SYNC: DisconnectSyncPulse.Rest" {
          n75 = Unbundle By Name(w312) -> ("Rest.TimeSync.Ref"=w310:refnum<k15>, "Rest.Sync Pulse.PFI --> Sync Pulse Source"=w307:T4)
          n76 = call-poly "Trigger_Poly.vi"("Routing Information"=w307, "instrument handle"=w310) -> ("error out"=w305:errorcluster, "instrument handle out"=w309:refnum<k15>)  [unwired: 8 in]
          n77 = Bundle By Name(cluster=w312, "Rest.TimeSync.Ref"=w309) -> (w311:T8)
          n78 = Merge Errors(w306, w305) -> (w304:errorcluster)
        }
        frame "SYNC: ConnectStartTrigger.Master" {
          n79 = Unbundle By Name(w321) -> ("Master.TimeSync.Ref"=w319:refnum<k15>, "Master.Start Trigger.Start Trigger --> PFI"=w314:T4)
          n80 = call-poly "Trigger_Poly.vi"("error in (no error)"=w316, "Routing Information"=w314, "instrument handle"=w319) -> ("error out"=w317:errorcluster, "instrument handle out"=w318:refnum<k15>)  [unwired: 7 in]
          n81 = Bundle By Name(cluster=w321, "Master.TimeSync.Ref"=w318) -> (w320:T8)
        }
        frame "SYNC: ConnectStartTrigger.Rest" {
          n82 = Unbundle By Name(w330) -> ("Rest.TimeSync.Ref"=w328:refnum<k15>, "Rest.Start Trigger.PFI --> Start Trigger"=w323:T4)
          n83 = call-poly "Trigger_Poly.vi"("error in (no error)"=w325, "Routing Information"=w323, "instrument handle"=w328) -> ("error out"=w326:errorcluster, "instrument handle out"=w327:refnum<k15>)  [unwired: 7 in]
          n84 = Bundle By Name(cluster=w330, "Rest.TimeSync.Ref"=w327) -> (w329:T8)
        }
        frame "TCLK: Commit" {
          n85 = Unbundle By Name(w335) -> ("Master.TCLK.Ref"=w337:refnum<k20>, "Rest.TCLK.Refs"=w336:refnum<k20>[])
          n86 = Build Array (concatenate)(w337, w336) -> (w334:refnum<k20>[])
          n87 = call <instrlib>:"niTClk Initiate.vi"("error in (no error)"=w333, "sessions"=w334) -> ("error out"=w332:errorcluster)  [unwired: 8 in, 1 out]
        }
        frame "FGEN: StartSquareWave" {
          w352 = u16 1 items=["Sine", "Square", "Triangle", "Ramp Up", "Ramp Down", "DC", "Noise"] ("Standard Waveform")
          w350 = T11 0 items=["Standard Function", "Frequency List", "Arbitrary Waveform", "Arbitrary Sequence", "Script"] ("output mode")
          n88 = Multiply(x=2.0, y=w342) -> (x*y=w341:dbl)
          n89 = call <instrlib>:"niFgen Initialize With Channels.vi"("error in (no error)"=w349, "Reset Device (default: False)"=TRUE, "Channel Name"="0", "Resource Name"=refnum<k15> "PXI1_FGEN1" ("FGEN Resource Name")) -> ("error out"=w360:errorcluster, "Instrument Handle Out"=w359:refnum<k15>)  [unwired: 6 in]
          n90 = call <instrlib>:"niFgen Configure Output Mode.vi"("error in (no error)"=w360, "Output Mode (default: 0=Standard Function)"=w350, "Instrument Handle"=w359) -> ("error out"=w358:errorcluster, "Instrument Handle Out"=w357:refnum<k15>)  [unwired: 6 in]
          n91 = call <instrlib>:"niFgen Configure Standard Waveform.vi"("Instrument Handle"=w357, "Waveform"=w352, "Frequency"=10000.0, "Amplitude"=w341, "error in (no error)"=w358) -> ("Instrument Handle Out"=w356:refnum<k15>, "error out"=w355:errorcluster)  [unwired: 9 in]
          n92 = call <instrlib>:"niFgen Initiate Generation.vi"("error in (no error)"=w355, "Instrument Handle"=w356) -> ("error out"=w348:errorcluster, "Instrument Handle Out"=w345:refnum<k15>)  [unwired: 8 in]
          n93 = Bundle By Name(cluster=w346, "FGEN.Ref"=w345) -> (w344:T8)
        }
        frame "SCOPE: Acquire" {
          n94 = Unbundle By Name(w377) -> ("Master.Scope.Ref"=w375:refnum<k15>, "Rest.Scope.Refs"=w376:refnum<k15>[])
          n95 = Build Array (concatenate)(w375, w376) -> (w373:refnum<k15>[])
          n96 = Array Size(array=w373) -> (size(s)=w372:i32)
          n97 = for {
            tunnel: w373 -> [w387] mode=indexing
            tunnel: [w382] -> w367 mode=indexing
            tunnel: w379 -> [w386]
            tunnel: [w390] -> w378 mode=indexing
            workers-P: w372 -> [_]
            tunnel: w366 -> [w381]
            w383 = 477 items=["Start"=482, "Trigger"=483, "Pretrigger"=477, "Now"=481, "Read Pointer"=388] ("Fetch:Fetch Relative To")
            n98 = property class="niScope"(reference=w387, error in=w386, "Fetch:Fetch Relative To"=w383) -> (reference out=w384:refnum<k15>, error out=w385:errorcluster)
            n99 = call-poly <instrlib>:"niScope Fetch (poly).vi"("timeout"=10.0, "error in"=w385, "numSamples"=w381, "channels"="0", "instrument handle"=w384) -> ("error out"=w390:errorcluster, "waveform"=w382:T12)  [unwired: 3 in, 2 out]
          }
          "Waveform Graph" <- w367
          n100 = Reciprocal(x=w365) -> (1/x=w363:dbl)
          n101 = Merge Errors(w378) -> (w374:errorcluster)
          n102 = Index Array(array=w367) -> (element #1=w371:T12, element #2=w370:T12)  [unwired: 2 in]
          n103 = Unbundle By Name(w371) -> ("wfm"=w368:dbl[])
          n104 = Unbundle By Name(w370) -> ("wfm"=w369:dbl[])
          n105 = call "Find Delta Samples of Rising Edge_DBL.vi"("Trigger Level"=w362, "Channel 2"=w369, "Channel 1"=w368) -> ("Sample Offset"=w364:dbl)  [unwired: 8 in]
          "Sample Offset" <- w364
          n106 = Multiply(x=w363, y=w364) -> (x*y=w361:dbl)
          "Offset Time (s)" <- w361
        }
        frame "FGEN: StopSquareWave" {
          n107 = Unbundle By Name(w397) -> ("FGEN.Ref"=w396:refnum<k15>)
          n108 = call <instrlib>:"niFgen Abort Generation.vi"("Instrument Handle"=w396) -> ("error out"=w399:errorcluster, "Instrument Handle Out"=w398:refnum<k15>)  [unwired: 9 in]
          n109 = call <instrlib>:"niFgen Close.vi"("error in (no error)"=w399, "Instrument Handle"=w398) -> ("error out"=w395:errorcluster)  [unwired: 9 in]
          n110 = Merge Errors(w394, w395) -> (w393:errorcluster)
        }
        frame "SYNC: DisconnectStartTrigger.Master" {
          n111 = Unbundle By Name(w409) -> ("Master.TimeSync.Ref"=w407:refnum<k15>, "Master.Start Trigger.Start Trigger --> PFI"=w403:T4)
          n112 = call-poly "Trigger_Poly.vi"("Routing Information"=w403, "instrument handle"=w407) -> ("error out"=w405:errorcluster, "instrument handle out"=w406:refnum<k15>)  [unwired: 8 in]
          n113 = Bundle By Name(cluster=w409, "Master.TimeSync.Ref"=w406) -> (w408:T8)
          n114 = Merge Errors(w401, w405) -> (w402:errorcluster)
        }
        frame "SYNC: DisconnectStartTrigger.Rest" {
          n115 = Unbundle By Name(w419) -> ("Rest.TimeSync.Ref"=w417:refnum<k15>, "Rest.Start Trigger.PFI --> Start Trigger"=w414:T4)
          n116 = call-poly "Trigger_Poly.vi"("Routing Information"=w414, "instrument handle"=w417) -> ("error out"=w412:errorcluster, "instrument handle out"=w416:refnum<k15>)  [unwired: 8 in]
          n117 = Bundle By Name(cluster=w419, "Rest.TimeSync.Ref"=w416) -> (w418:T8)
          n118 = Merge Errors(w411, w412) -> (w413:errorcluster)
        }
        frame "SYNC: DisconnectRefTrigger.Master" {
          n119 = Unbundle By Name(w429) -> ("Master.TimeSync.Ref"=w427:refnum<k15>, "Master.Ref Trigger.Ref Trigger --> PFI"=w424:T4)
          n120 = call-poly "Trigger_Poly.vi"("Routing Information"=w424, "instrument handle"=w427) -> ("error out"=w422:errorcluster, "instrument handle out"=w426:refnum<k15>)  [unwired: 8 in]
          n121 = Bundle By Name(cluster=w429, "Master.TimeSync.Ref"=w426) -> (w428:T8)
          n122 = Merge Errors(w423, w422) -> (w421:errorcluster)
        }
        frame "SYNC: DisconnectRefTrigger.Rest" {
          n123 = Unbundle By Name(w439) -> ("Rest.TimeSync.Ref"=w437:refnum<k15>, "Rest.Ref Trigger.PFI --> Ref Trigger"=w434:T4)
          n124 = call-poly "Trigger_Poly.vi"("Routing Information"=w434, "instrument handle"=w437) -> ("error out"=w433:errorcluster, "instrument handle out"=w436:refnum<k15>)  [unwired: 8 in]
          n125 = Bundle By Name(cluster=w439, "Rest.TimeSync.Ref"=w436) -> (w438:T8)
          n126 = Merge Errors(w431, w433) -> (w432:errorcluster)
        }
        frame "SYNC: DisconnectClock.Master" {
          n127 = Unbundle By Name(w451) -> ("Master.TimeSync.Ref"=w449:refnum<k15>, "Master.Clock.Clock --> Out"=w447:T3, "Master.Clock.In --> Clk10"=w446:T3)
          n128 = Build Array(w447, w446) -> (w445:T3[])
          n129 = call-poly "Clock_Poly.vi"("Clock Routing"=w445, "instrument handle"=w449) -> ("error out"=w441:errorcluster, "instrument handle out"=w448:refnum<k15>)  [unwired: 8 in]
          n130 = Bundle By Name(cluster=w451, "Master.TimeSync.Ref"=w448) -> (w450:T8)
          n131 = Merge Errors(w443, w441) -> (w442:errorcluster)
        }
        frame "SYNC: DisconnectClock.Rest" {
          n132 = Unbundle By Name(w461) -> ("Rest.TimeSync.Ref"=w459:refnum<k15>, "Rest.Clock.In --> Clk10"=w456:T3)
          n133 = call-poly "Clock_Poly.vi"("Clock Routing"=w456, "instrument handle"=w459) -> ("error out"=w453:errorcluster, "instrument handle out"=w458:refnum<k15>)  [unwired: 8 in]
          n134 = Bundle By Name(cluster=w461, "Rest.TimeSync.Ref"=w458) -> (w460:T8)
          n135 = Merge Errors(w455, w453) -> (w454:errorcluster)
        }
        frame "Shutdown" {
          n136 = Unbundle By Name(w475) -> ("Master.TimeSync.Ref"=w474:refnum<k15>, "Rest.TimeSync.Ref"=w473:refnum<k15>, "Master.Scope.Ref"=w472:refnum<k15>, "Rest.Scope.Refs"=w471:refnum<k15>[])
          n137 = Build Array(w474, w473) -> (w469:refnum<k15>[])
          n138 = Build Array (concatenate)(w472, w471) -> (w470:refnum<k15>[])
          n139 = for {
            tunnel: w469 -> [w477] mode=indexing
            tunnel: [w476] -> w466 mode=indexing
            n140 = call <instrlib>:"niSync Close.vi"("instrument handle"=w477) -> ("error out"=w476:errorcluster)  [unwired: 10 in]
          }
          n141 = for {
            tunnel: w470 -> [w479] mode=indexing
            tunnel: [w478] -> w467 mode=indexing
            n142 = call <instrlib>:"niScope Close.vi"("instrument handle"=w479) -> ("error out"=w478:errorcluster)  [unwired: 14 in]
          }
          n143 = Merge Errors(w468, w467, w466) -> (w465:errorcluster)
        }
      }
      n144 = Increment(x=w38) -> (x+1=w36:T7)
    }
    n145 = Unbundle By Name(w13) -> ("status"=w12:bool)
    n146 = Not(x=w12) -> (.not. x?=w11:bool)
  }
  "Cal Iteration Delays" <- w3
  n147 = for {
    tunnel: w3 -> [w484] mode=indexing
    tunnel: [w483] -> w1
    tunnel: [w482] -> w2
    i -> [w481]
    n148 = Equal To 0?(x=w481) -> (x = 0?=w480:bool)
    n149 = call <vilib>:"Standard Deviation PtByPt.vi"("x"=w484, "initialize"=w480) -> ("standard deviation"=w483:dbl, "mean"=w482:dbl)  [unwired: 1 in, 1 out]
  }
  "Average Delay" <- w2
  "Standard Deviation" <- w1
  n150 = call <vilib>:"Simple Error Handler.vi"("error in (no error)"=w9) -> ("error out"=→"error out":errorcluster)  [unwired: 4 in, 4 out]
